vi "Z eq CELL (SubVI).vi"(1 "Rcycle":dbl, 2 "SOC":dbl) -> (0 "Z eq CELL":dbl)   [LabVIEW 2017]
panel:
  out "C transient_L":dbl
  out "R  transient_L":dbl
  out "C transient_s":dbl
  out "R transient_s":dbl
  out "R series":dbl
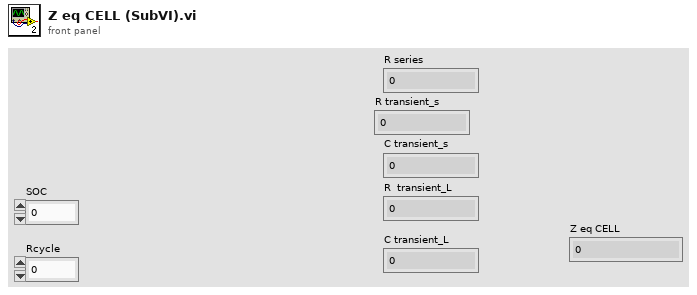
[diagram p1: front panel]
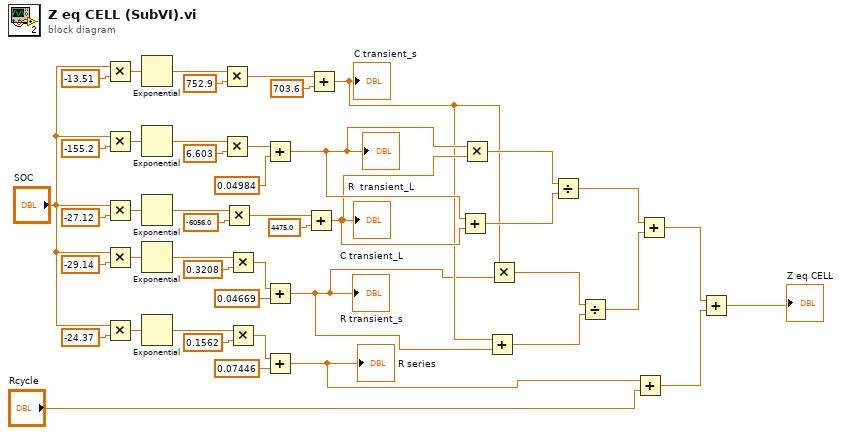
[diagram p0: block diagram]
diagram:
  n1 = Multiply(x="SOC", y=-13.51) -> (x*y=w33:dbl)
  n2 = Multiply(x="SOC", y=-155.2) -> (x*y=w27:dbl)
  n3 = Multiply(x="SOC", y=-27.12) -> (x*y=w21:dbl)
  n4 = Multiply(x="SOC", y=-29.14) -> (x*y=w39:dbl)
  n5 = Multiply(x="SOC", y=-24.37) -> (x*y=w45:dbl)
  n6 = Exponential(1:w33) -> (0:w32:dbl)
  n7 = Exponential(1:w27) -> (0:w26:dbl)
  n8 = Exponential(1:w21) -> (0:w20:dbl)
  n9 = Exponential(1:w39) -> (0:w38:dbl)
  n10 = Exponential(1:w45) -> (0:w44:dbl)
  n11 = Multiply(x=w32, y=752.9) -> (x*y=w30:dbl)
  n12 = Multiply(x=w26, y=6.603) -> (x*y=w24:dbl)
  n13 = Multiply(x=w20, y=-6056.0) -> (x*y=w18:dbl)
  n14 = Multiply(x=w38, y=0.3208) -> (x*y=w36:dbl)
  n15 = Multiply(x=w44, y=0.1562) -> (x*y=w42:dbl)
  n16 = Add(x=w24, y=0.04984) -> (x+y=w15:dbl)
  "R  transient_L" <- w15
  n17 = Add(x=w36, y=0.04669) -> (x+y=w8:dbl)
  "R transient_s" <- w8
  n18 = Add(x=w42, y=0.07446) -> (x+y=w5:dbl)
  "R series" <- w5
  n19 = Add(x=w18, y=4475.0) -> (x+y=w14:dbl)
  "C transient_L" <- w14
  n20 = Add(x=w30, y=703.6) -> (x+y=w9:dbl)
  "C transient_s" <- w9
  n21 = Add(x=w15, y=w14) -> (x+y=w13:dbl)
  n22 = Multiply(x=w15, y=w14) -> (x*y=w12:dbl)
  n23 = Add(x=w9, y=w8) -> (x+y=w11:dbl)
  n24 = Multiply(x=w9, y=w8) -> (x*y=w10:dbl)
  n25 = Divide(x=w12, y=w13) -> (x/y=w7:dbl)
  n26 = Divide(x=w10, y=w11) -> (x/y=w6:dbl)
  n27 = Add(x=w5, y="Rcycle") -> (x+y=w2:dbl)
  n28 = Add(x=w7, y=w6) -> (x+y=w3:dbl)
  n29 = Add(x=w3, y=w2) -> (x+y=→"Z eq CELL":dbl)
